vi "calculateDeltaTimestamp.vi"(8 "error in (no error)":errorcluster, 11 "TrapezoidalWave in":refnum<class "TrapezoidalWave.lvclass">) -> (0 "error out":errorcluster, 2 "Delta Timestamp":dbl format="%.9f", 3 "TrapezoidalWave out":refnum<class "TrapezoidalWave.lvclass">)   [LabVIEW 2015, in "TrapezoidalWave.lvclass"]
uses:
  TrapezoidalWave.lvclass
  TrapezoidalWave.lvclass/TrapezoidalWave.ctl
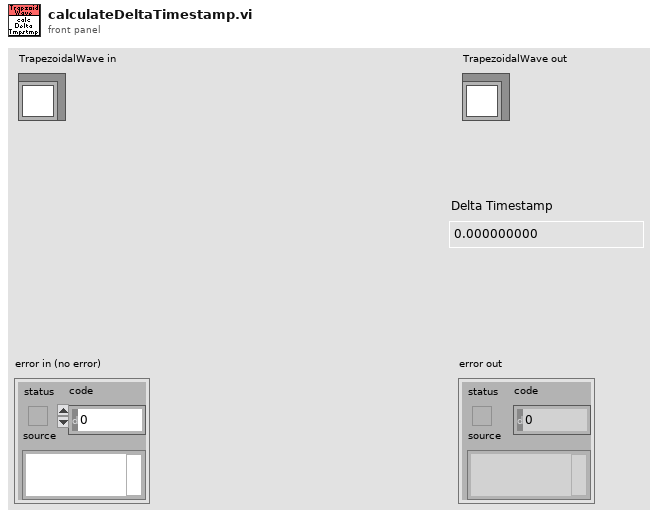
[diagram p1: front panel]
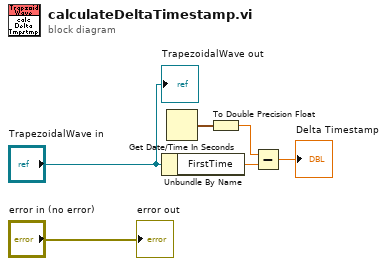
[diagram p0: block diagram]
diagram:
  n1 = Unbundle By Name("TrapezoidalWave in") -> ("FirstTime"=w3:dbl)
  n2 = Get Date/Time In Seconds() -> (seconds since 1Jan1904=w1:timestamp)
  n3 = To Double Precision Float(number=w1) -> (double precision float=w5:dbl)
  n4 = Subtract(x=w5, y=w3) -> (x-y=→"Delta Timestamp":dbl)
  "error out" <- "error in (no error)"
  "TrapezoidalWave out" <- "TrapezoidalWave in"
